vi "Limelight_Differential.vi"() -> (0 "TargetValid":bool, 2 "SteerCommand":dbl(knob)=nan scale=-1.0..1.0, 3 "DriveCommand":dbl(knob)=-0.0 scale=-1.0..1.0)   [LabVIEW 2020]
uses:
  <vilib>/Rock Robotics/Network Tables/NT Read Number.vi
  Framework/Robot Global Data.vi
panel:
  out "MaxDrive":dbl(slide)=0.6824817518248175 min=0.0 max=1.0 step=0.01 scale=0.0..1.0
  out "DriveK":dbl(slide)=0.26277372262773724 min=0.0 max=1.0 step=0.05 scale=0.0..1.0
  out "Limelight Goal Area":dbl(slide)=14.8723 min=0.1 max=25.0 step=0.25 scale=0.0..25.0
  out "AimDeadband":dbl min=0.0 max=10.0 step=0.25
  out "MinSteerCommand":dbl(slide)=0.2717391304347826 min=0.0 max=0.5 step=0.05 scale=0.0..0.5
  out "SteeringK":dbl(slide)=0.025362318840579712 min=0.0 max=0.25 step=0.01 scale=0.0..0.25
  # "0.0253623"
  # "0.271739"
  # "14.8723"
  # "0.262774"
  # "0.682482"
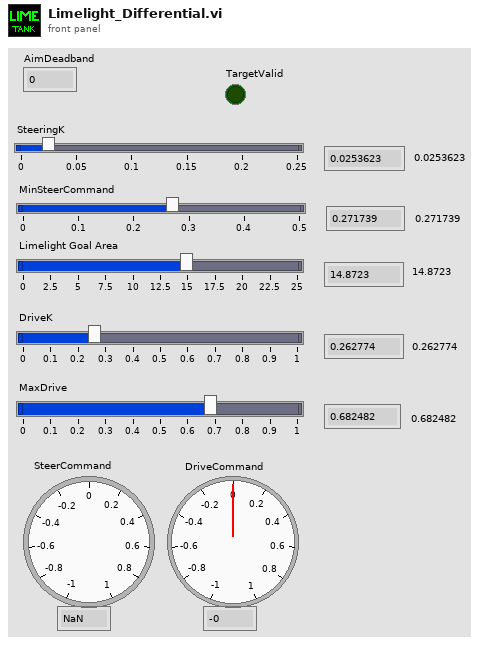
[diagram p1: front panel]
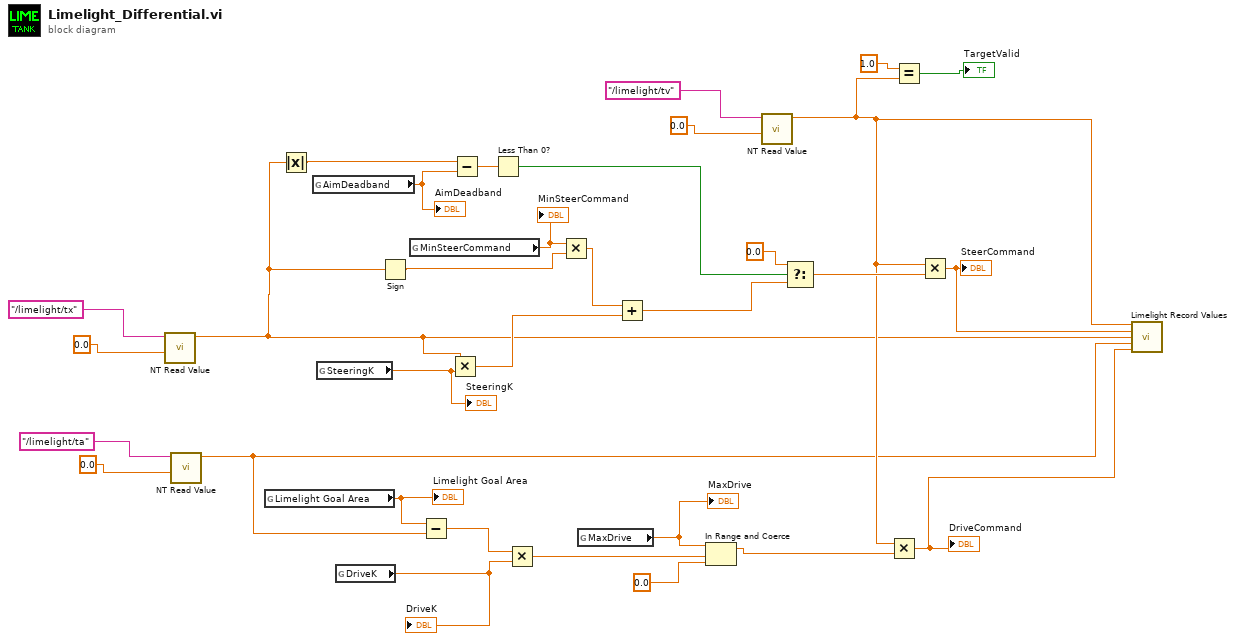
[diagram p0: block diagram]
diagram:
  n1 = call-poly <vilib>:"NT Read Value.vi"("Default Value"=0.0, "Name"="/limelight/tx") -> ("Numeric"=w3:dbl)  [unwired: 8 in, 1 out]
  n2 = call-poly <vilib>:"NT Read Value.vi"("Default Value"=0.0, "Name"="/limelight/ta") -> ("Numeric"=w2:dbl)  [unwired: 8 in, 1 out]
  n3 = global read "Robot Global Data.vi" "Limelight Goal Area"() -> (w8:dbl)
  "Limelight Goal Area" <- w8
  n4 = Absolute Value(x=w3) -> (abs(x)=w29:dbl)
  n5 = global read "Robot Global Data.vi" "AimDeadband"() -> (w11:dbl)
  "AimDeadband" <- w11
  n6 = global read "Robot Global Data.vi" "SteeringK"() -> (w9:dbl)
  "SteeringK" <- w9
  n7 = global read "Robot Global Data.vi" "DriveK"() -> (w6:dbl)
  "DriveK" <- w6
  n8 = Sign(1:w3) -> (0:w19:dbl)
  n9 = global read "Robot Global Data.vi" "MinSteerCommand"() -> (w10:dbl)
  "MinSteerCommand" <- w10
  n10 = Subtract(x=w8, y=w2) -> (x-y=w18:dbl)
  n11 = Multiply(x=w3, y=w9) -> (x*y=w27:dbl)
  n12 = Subtract(x=w29, y=w11) -> (x-y=w30:dbl)
  n13 = Less Than 0?(x=w30) -> (x < 0?=w31:bool)
  n14 = Multiply(x=w18, y=w6) -> (x*y=w17:dbl)
  n15 = Multiply(x=w10, y=w19) -> (x*y=w28:dbl)
  n16 = global read "Robot Global Data.vi" "MaxDrive"() -> (w7:dbl)
  "MaxDrive" <- w7
  n17 = Add(x=w28, y=w27) -> (x+y=w14:dbl)
  n18 = In Range and Coerce(upper limit=w7, x=w17, lower limit=0.0) -> (coerced(x)=w15:dbl)  [unwired: 1 out]
  n19 = call-poly <vilib>:"NT Read Value.vi"("Default Value"=0.0, "Name"="/limelight/tv") -> ("Numeric"=w5:dbl)  [unwired: 8 in, 1 out]
  n20 = Select(t=0.0, s=w31, f=w14) -> (s? t:f=w20:dbl)
  n21 = Multiply(x=w5, y=w15) -> (x*y=w1:dbl)
  "DriveCommand" <- w1
  n22 = Equal?(x=1.0, y=w5) -> (x = y?=→"TargetValid":bool)
  n23 = Multiply(x=w5, y=w20) -> (x*y=w4:dbl)
  "SteerCommand" <- w4
  n24 = call "Limelight Record Values.vi"("tv"=w5, "Steer"=w4, "tx"=w3, "ta"=w2, "Drive"=w1) -> ()  [unwired: 11 in]
